vi "IndexStepsArray.vi"(9 "index":i32, 11 "Steps Array":T2[](array[typedef])) -> (1 "Previus":T1=enum."Idle", 3 "Index out":i32)   [LabVIEW 2019]
doc: "Controlla se l'index è minore della lunghezza dell'array e imposta lo stato successivo"
uses:
  TypeDef/StepSimulationInfo.ctl
  TypeDef/SimulatoreStates.ctl
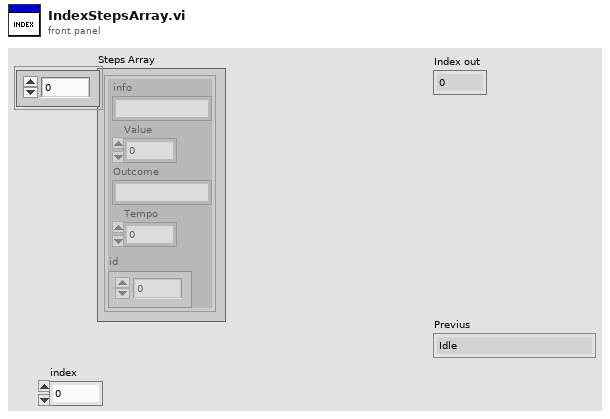
[diagram p1: front panel]
types:
  T1 = typedef "SimulatoreStates.ctl" = enum16{"Initialize", "Idle", "GetLimsTestsForBench", "GetLimsTestSteps", "Simulation Start", "WaitForLigths"}
  T2 = typedef "StepSimulationInfo.ctl" = cluster{"info":string, "Value":dbl, "Outcome":string, "Tempo":dbl, "id":dbl}
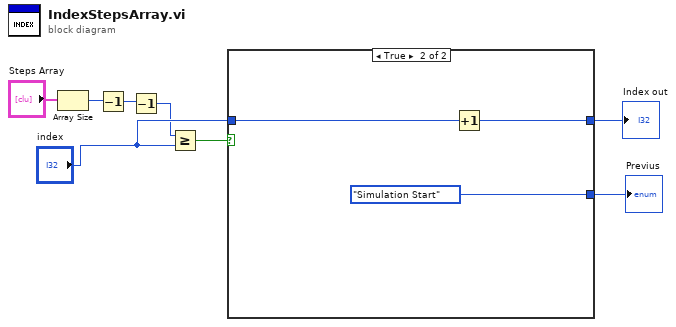
[diagram p0: block diagram]
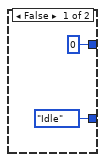
[diagram p2: hidden frame]
diagram:
  n1 = Array Size(array="Steps Array") -> (size(s)=w7:i32)
  n2 = Decrement(x=w7) -> (x-1=w2:i32)
  n3 = Decrement(x=w2) -> (x-1=w1:i32)
  n4 = Greater Or Equal?(x=w1, y="index") -> (x >= y?=w6:bool)
  n5 = case shown="True" w6 {
    tunnel: "index" -> [_ w13]
    tunnel: [0 w12] -> w4
    tunnel: [SimulatoreStates."Idle" ("Previus") SimulatoreStates."Simulation Start" ("Previus")] -> w3
    frame False {
    }
    frame True {
      n6 = Increment(x=w13) -> (x+1=w12:i32)
    }
  }
  "Index out" <- w4
  "Previus" <- w3
